vi "Write Log Column Header.vi"(8 "error in (no error)":errorcluster, 11 "Model in":refnum<class "Model.lvclass">) -> (0 "error out":errorcluster, 3 "Model out":refnum<class "Model.lvclass">)   [LabVIEW 2015, in "Model.lvclass"]
uses:
  Model.lvclass
  Model.lvclass/Model.ctl
  Test Log/Test Log/Test Log.lvclass
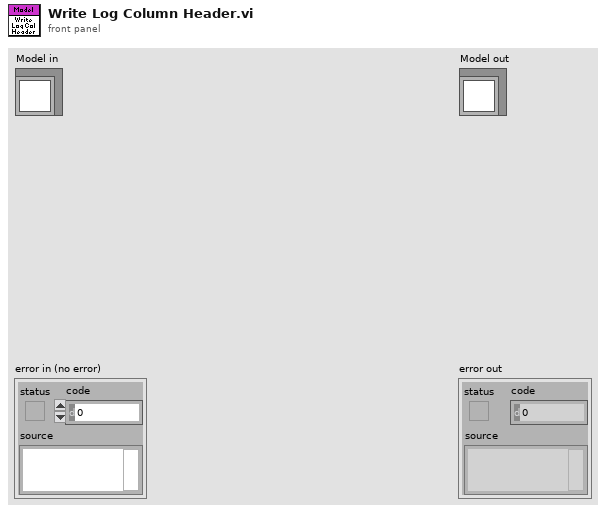
[diagram p1: front panel]
types:
  T1 = typedef "FAMT Typedefs.lvlib/Actuator Types.ctl" = enum16{"Single", "Dual"}
  T2 = typedef "FAMT Typedefs.lvlib/Cylinder Types.ctl" = enum16{"PSV Open", "PSV Closed", "TV Open", "TV Closed", "Closed"}
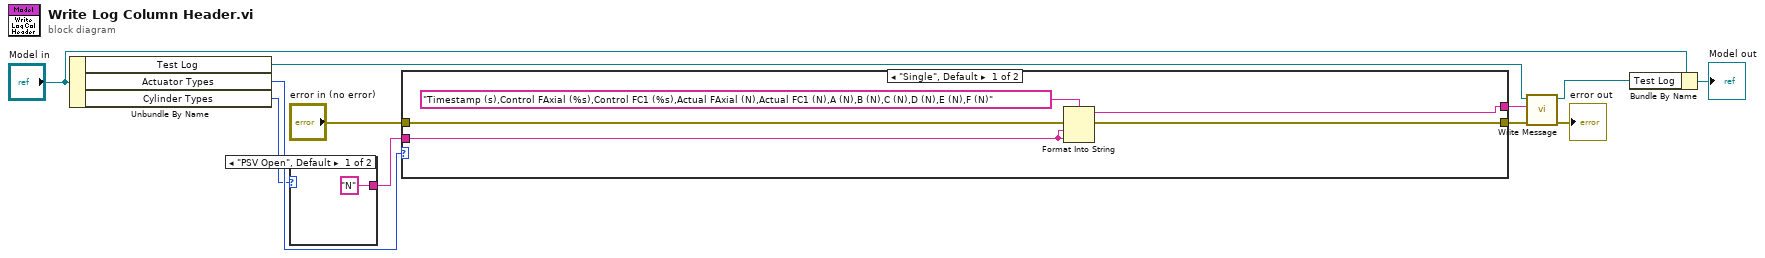
[diagram p0: block diagram]
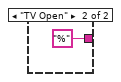
[diagram p2: hidden frame]
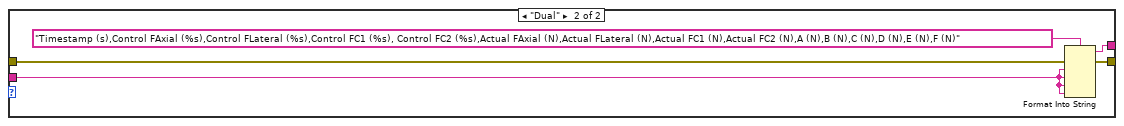
[diagram p3: hidden frame]
diagram:
  n1 = Unbundle By Name("Model in") -> ("Test Log"=w1:refnum<class "Test Log.lvclass">, "Actuator Types"=w9:T1, "Cylinder Types"=w8:T2)
  n2 = case shown="\"PSV Open\", Default" w8 {
    tunnel: ["N" "%"] -> w7
    frame "PSV Open", Default {
    }
    frame "TV Open" {
    }
  }
  n3 = case shown="\"Single\", Default" w9 {
    tunnel: [w14 w19] -> w5
    tunnel: w7 -> [w17 w22]
    tunnel: "error in (no error)" -> [w15 w21]
    tunnel: [w16 w20] -> w3
    frame "Single", Default {
      n4 = Format Into String(format string="Timestamp (s),Control FAxial (%s),Control FC1 (%s),Actual FAxial (N),Actual FC1 (N),A (N),B (N),C (N),D (N),E (N),F (N)", error in=w15, w17, w17) -> (resulting string=w14:string, error out=w16:errorcluster)  [unwired: 1 in]
    }
    frame "Dual" {
      n5 = Format Into String(format string="Timestamp (s),Control FAxial (%s),Control FLateral (%s),Control FC1 (%s), Control FC2 (%s),Actual FAxial (N),Actual FLateral (N),Actual FC1 (N),Actual FC2 (N),A (N),B (N),C (N),D (N),E (N),F (N)", error in=w21, w22, w22, w22, w22) -> (resulting string=w19:string, error out=w20:errorcluster)  [unwired: 1 in]
    }
  }
  n6 = call-dynamic "Write Message.vi"("error in (no error)"=w3, "Message"=w5, "Test Log in"=w1) -> ("error out"=→"error out":errorcluster, "Test Log out"=w4:refnum<class "Test Log.lvclass">)  [unwired: 7 in]
  n7 = Bundle By Name(cluster="Model in", "Test Log"=w4) -> (→"Model out":refnum<class "Model.lvclass">)
